vi "ASM.Settings.AutoContinue.vi"(8 "error in (no error)":errorcluster, 10 "AutoContinue":bool, 11 "ActorStateMachine in":refnum<class "ActorStateMachine.lvclass">) -> (0 "error out":errorcluster, 3 "ActorStateMachine out":refnum<class "ActorStateMachine.lvclass">)   [LabVIEW 2021, in "ActorStateMachine.lvlib" / "ActorStateMachine.lvclass"]
uses:
  ActorStateMachine.lvclass
  ActorStateMachine.lvclass/ActorStateMachine.ctl
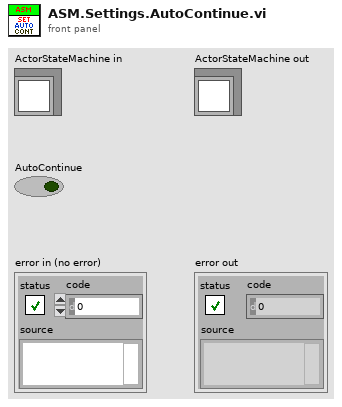
[diagram p1: front panel]
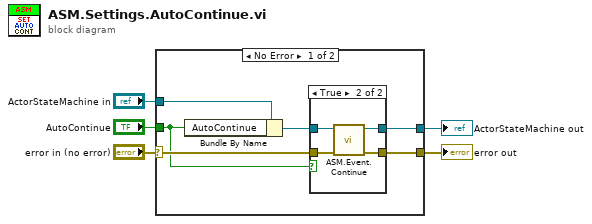
[diagram p0: block diagram]
diagram:
  n1 = case shown="No Error" "error in (no error)" {
    selector: "error in (no error)" -> [w8 w19]
    tunnel: [w7 w19] -> w4
    tunnel: [w9 w18] -> w2
    tunnel: "ActorStateMachine in" -> [w11 w18]
    tunnel: "AutoContinue" -> [w6 _]
    frame No Error {
      n2 = Bundle By Name(cluster=w11, "AutoContinue"=w6) -> (w10:refnum<class "ActorStateMachine.lvclass">)
      n3 = case shown="True" w6 {
        tunnel: w10 -> [w13 w17]
        tunnel: [w13 w16] -> w9
        tunnel: w8 -> [w12 w15]
        tunnel: [w12 w14] -> w7
        frame False {
        }
        frame True {
          n4 = call "ASM.Event.Continue.vi"("error in (no error)"=w15, "ActorStateMachine in"=w17) -> ("error out"=w14:errorcluster, "ActorStateMachine out"=w16:refnum<class "ActorStateMachine.lvclass">)  [unwired: 8 in]
        }
      }
    }
    frame Error {
    }
  }
  "error out" <- w4
  "ActorStateMachine out" <- w2
